vi "Camera Open.vi"(11 "command line":string="C:\\Runtime\\LightBoxAssembly\\Run Modified.exe") -> ()   [LabVIEW 2015]
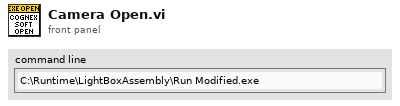
[diagram p1: front panel]
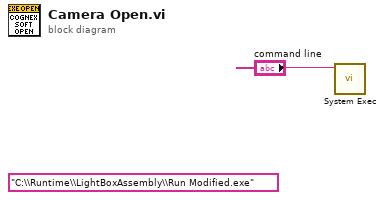
[diagram p0: block diagram]
diagram:
  (unwired) "C:\\Runtime\\LightBoxAssembly\\Run Modified.exe" ("command line")
  n1 = call <vilib>:"System Exec.vi"("command line"="command line") -> ()  [unwired: 7 in, 4 out]
